vi "pracownia3.vi"() -> ()   [LabVIEW 2019]
panel:
  out "y":string
  in  "Enum":T1(ring)
  in  "?":bool
  in  "?":bool
  in  "c":dbl
  in  "b":dbl
  in  "a":dbl
  in  "x":dbl
  # "y = a + bx + cx^2"
  # "y = a + bx^2 - 3x^4"
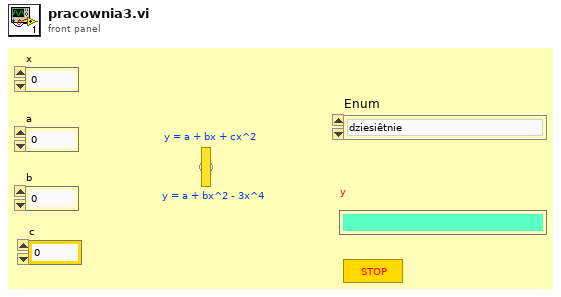
[diagram p1: front panel]
types:
  T1 = enum16{"dziesiêtnie ", "ósemkowo", "szesnastkowo"}
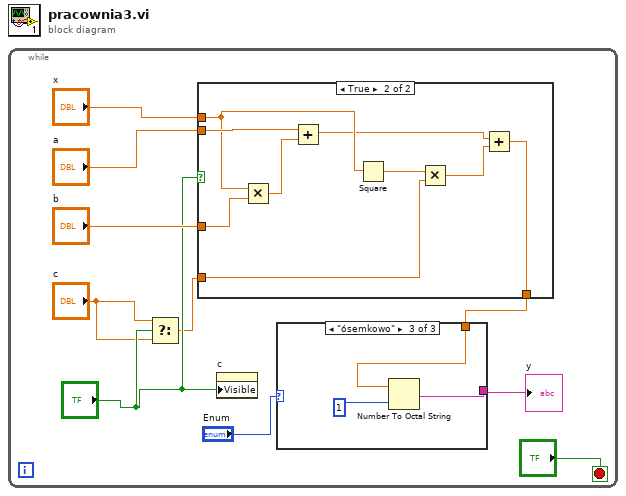
[diagram p0: block diagram]
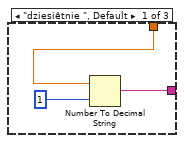
[diagram p2: hidden frame]
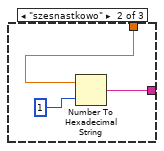
[diagram p3: hidden frame]
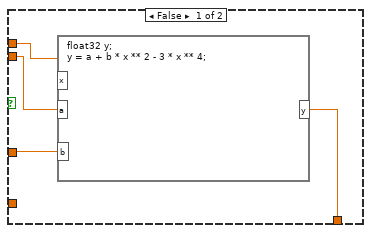
[diagram p4: hidden frame]
diagram:
  n1 = while {
    stop <- "?" stop-if-true
    n2 = Select(t="c", s="?", f="c") -> (s? t:f=w5:dbl)
    n3 = case shown="True" "?" {
      tunnel: "a" -> [w22 w32]
      tunnel: "x" -> [w23 w29]
      tunnel: "b" -> [w21 w31]
      tunnel: w5 -> [_ w28]
      tunnel: [w20 w24] -> w2
      frame False {
        n4 = formula code="float32 y;\ny = a + b * x ** 2 - 3 * x ** 4;"("x"=w23, "a"=w22, "b"=w21) -> ("y"=w20:sgl)
      }
      frame True {
        n5 = Multiply(x=w29, y=w31) -> (x*y=w30:dbl)
        n6 = Add(x=w32, y=w30) -> (x+y=w25:dbl)
        n7 = Square(x=w29) -> (x^2=w27:dbl)
        n8 = Multiply(x=w27, y=w28) -> (x*y=w26:dbl)
        n9 = Add(x=w25, y=w26) -> (x+y=w24:dbl)
      }
    }
    n10 = property on="c" class="DigNum (strict)"("Visible"="?") -> ()  [unwired: 2 in, 2 out]
    n11 = case shown="\"ósemkowo\"" "Enum" {
      tunnel: w2 -> [w13 w15 w18]
      tunnel: [w11 w16 w17] -> w1
      frame "dziesiêtnie ", Default {
        n12 = Number To Decimal String(number=w13, width (-)=i16 1) -> (decimal integer string=w11:string)
      }
      frame "szesnastkowo" {
        n13 = Number To Hexadecimal String(1:1, 2:w15) -> (0:w16:string)
      }
      frame "ósemkowo" {
        n14 = Number To Octal String(1:1, 2:w18) -> (0:w17:string)
      }
    }
    "y" <- w1
  }
